vi "simple_strain_test.vi"() -> ()   [LabVIEW 2013]
uses:
  ctl/force_sensor_data.ctl
  ctl/strain_ctl.ctl
  <vilib>/Analysis/baseanly.llb/Mean (DBL).vi
  Global.vi
  <vilib>/Waveform/WDTFileIO.llb/ Write Waveform to File.vi
  <vilib>/Analysis/NI_AALBase.lvlib
panel:
  in  "정지":bool
  in  "탭 컨트롤 2":enum32{"페이지 1", "페이지 2"}(tab)
  out "ratio chart":T1(graph)
  out "balance ok":bool
  out "balance graph":T2(graph)
  out "Force Graph":waveform(dbl)[](graph)
  out "p 4":dbl format="%.2f"
  out "p 3":dbl format="%.2f"
  out "p 2":dbl format="%.2f"
  out "p 1":dbl format="%.2f"
  out "chart":dbl(graph)
  out "출력 클러스터":T3 {"mean" format="%.6f"; "mean" format="%.6f"; "mean" format="%.6f"; "mean" format="%.6f"}
  in  "cal":bool
  out "strain sum 2":dbl format="%.6f"
  out "strain sum1":dbl format="%.6f"
  out "g weight":dbl format="%0.2f"
  out "portion ok":bool
  in  "balance update":bool
  out "웨이브폼 그래프":dbl[][](graph)
  out "error out 2":errorcluster caption="error out"
  in  "Force Sensor data":T4 {"strain map"."x" format="%#.7f"}
  in  "write\nforce data":bool
  in  "탭 컨트롤":enum32{"페이지 1", "페이지 2"}(tab)
  in  "file path (dialog if empty)":path caption="파일 경로(비었을 경우 대화 상자 창)"
  out "숫자형":i32
  in  "save?":bool
  in  "filter":bool
  in  "Lower Cut-Off":dbl=100.0 caption="하위 컷오프"
  out "Strain_offset_data":waveform(dbl)[](array[waveform])
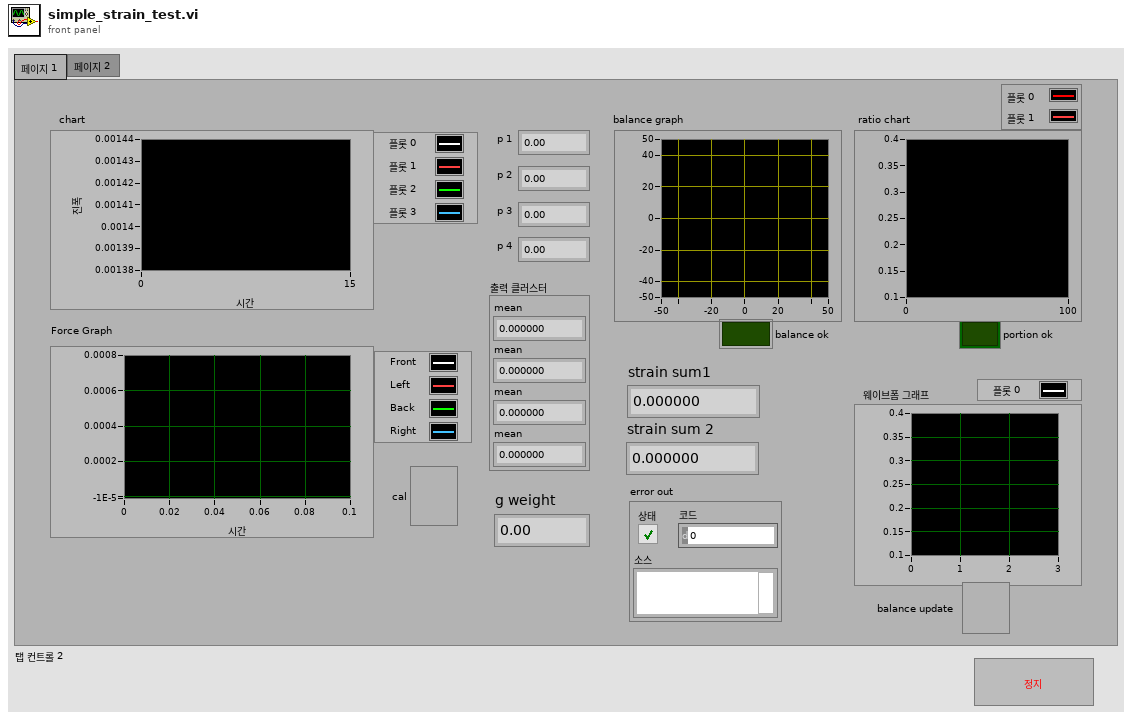
[diagram p1: front panel]
types:
  T1 = cluster{"[0]":dbl, "[1]":dbl, "[2]":dbl, "[3]":dbl, "[4]":dbl, "[5]":dbl, "[6]":dbl, "[7]":dbl, "[8]":dbl}
  T2 = cluster{"Balance xy wfs":cluster{"X":dbl, "Y":dbl}[]}[]
  T3 = cluster{"mean":dbl, "mean":dbl, "mean":dbl, "mean":dbl}
  T4 = typedef "force_sensor_data.ctl" = cluster{"weight":cluster{"front":dbl, "left":dbl, "back":dbl, "right":dbl}, "strain map":cluster{"x":dbl, "y":dbl}[]}
  T5 = typedef "strain_ctl.ctl" = enum16{"config", "start", "read", "close"}
  T6 = cluster{"Balance xy wfs":cluster{"X":dbl, "Y":dbl}[]}
  T7 = cluster{"[0]":dbl, "[1]":dbl, "[2]":dbl, "[3]":dbl}
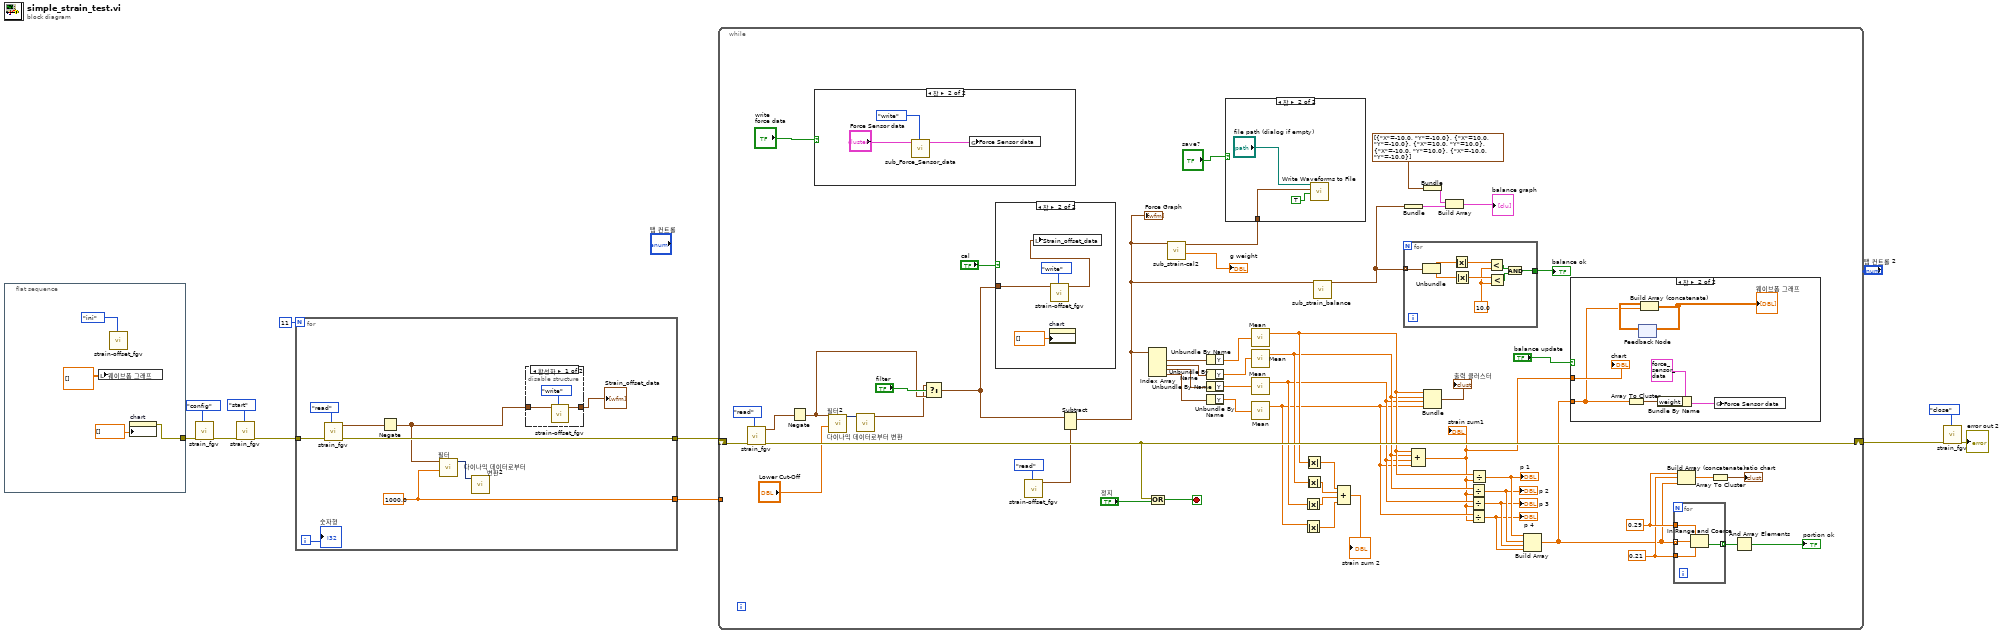
[diagram p0: block diagram]
diagram:
  n1 = flat-sequence {
    tunnel: [w15] -> w3
    frame #0 {
      n2 = local write "웨이브폼 그래프"(dbl[][] [] ("웨이브폼 그래프")) -> ()
      n3 = call "strain-offset_fgv.vi"("cmd"=enum16{"ini", "write", "read"}."ini") -> ()  [unwired: 9 in, 2 out]
      n4 = property on="chart" class="WFChart (엄격한)"("History Data"=dbl[] [] ("히스토리 데이터")) -> (error out=w15:errorcluster)  [unwired: 2 in, 1 out]
    }
  }
  n5 = call "strain_fgv.vi"("cmd"=strain_ctl."config", "error in"=w3) -> ("error out"=w7:errorcluster)  [unwired: 8 in, 1 out]
  n6 = call "strain_fgv.vi"("cmd"=strain_ctl."start", "error in"=w7) -> ("error out"=w6:errorcluster)  [unwired: 8 in, 1 out]
  n7 = for {
    N: 11 -> [_]
    tunnel: w6 -> [w24]
    tunnel: [w23] -> w5
    tunnel: [w20] -> w4
    i -> [w17]
    w20 = 1000.0 ("Lower Cut-Off")
    n8 = call "strain_fgv.vi"("cmd"=strain_ctl."read", "error in"=w24) -> ("error out"=w23:errorcluster, "data"=w21:waveform(dbl)[])  [unwired: 8 in]
    n9 = Negate(x=w21) -> (-x=w16:waveform(dbl)[])
    n10 = call "필터"("Lower Cut-Off"=w20, "Signal"=w16) -> ("Filtered Signal"=w22:dynamicdata)  [unwired: 8 in, 1 out]
    n11 = call "다이나믹 데이터로부터 변환2"("Dynamic Data Type"=w22) -> ()  [unwired: 3 in, 1 out]
    n12 = disable-structure shown="활성화" {
      disable-tunnel: w16 -> [w27 w28]
      disable-tunnel: [w26 w28] -> w19
      frame Enabled {
        n13 = call "strain-offset_fgv.vi"("cmd"=enum16{"ini", "write", "read"}."write", "data"=w27) -> ("Strain_offset_data"=w26:waveform(dbl)[])  [unwired: 8 in, 1 out]
      }
      frame Disabled {
      }
    }
    "Strain_offset_data" <- w19
    "숫자형" <- w17
  }
  n14 = while {
    shift-right: [w82] -> w11
    shift-left: w5 -> [w84]
    tunnel: w4 -> [_]
    stop <- w83 stop-if-true
    w37 = 0.21 ("하위 리미트")
    w38 = 0.29 ("하위 리미트")
    n15 = call "strain_fgv.vi"("cmd"=strain_ctl."read", "error in"=w84) -> ("error out"=w82:errorcluster, "data"=w69:waveform(dbl)[])  [unwired: 8 in]
    n16 = Negate(x=w69) -> (-x=w60:waveform(dbl)[])
    n17 = case shown="참" "write\nforce data" {
      frame False {
      }
      frame True {
        n18 = call "sub_Force_Sensor_data.vi"("cmd"=enum16{"write", "read"}."write", "Force Sensor data"="Force Sensor data") -> ("Force Sensor data out"=w107:T4)  [unwired: 9 in]
        n19 = global write "Global.vi" "Force Sensor data"(w107) -> ()
      }
    }
    n20 = call "필터2"("Lower Cut-Off"="Lower Cut-Off", "Signal"=w60) -> ("Filtered Signal"=w72:dynamicdata)  [unwired: 8 in, 1 out]
    n21 = call "다이나믹 데이터로부터 변환"("Dynamic Data Type"=w72) -> ("Array of Waveform"=w59:waveform(dbl)[])  [unwired: 3 in]
    n22 = Select(t=w59, s="filter", f=w60) -> (s? t:f=w63:waveform(dbl)[])
    n23 = case shown="참" "cal" {
      tunnel: w63 -> [_ w115]
      frame False {
      }
      frame True {
        n24 = property on="chart" class="WFChart (엄격한)"("History Data"=dbl[] [] ("히스토리 데이터")) -> ()  [unwired: 2 in, 2 out]
        n25 = call "strain-offset_fgv.vi"("cmd"=enum16{"ini", "write", "read"}."write", "data"=w115) -> ("Strain_offset_data"=w114:waveform(dbl)[])  [unwired: 8 in, 1 out]
        n26 = local write "Strain_offset_data"(w114) -> ()
      }
    }
    n27 = call "strain-offset_fgv.vi"("cmd"=enum16{"ini", "write", "read"}."read") -> ("Strain_offset_data"=w70:waveform(dbl)[])  [unwired: 9 in, 1 out]
    n28 = Subtract(1:w70, 2:w63) -> (0:w49:waveform(dbl)[])  [unwired: 1 in, 1 out]
    "Force Graph" <- w49
    n29 = Index Array(array=w49) -> (element #1=w80:waveform(dbl), element #2=w79:waveform(dbl), element #3=w78:waveform(dbl), element #4=w77:waveform(dbl))  [unwired: 4 in]
    n30 = Compound Arithmetic op=OR(w82, "정지") -> (w83:bool)
    n31 = call "sub_strain-cal2.vi"("strain wfs"=w49) -> ("force"=→"g weight":dbl, "force wf"=w65:waveform(dbl))  [unwired: 9 in]
    n32 = Unbundle By Name(w80) -> ("Y"=w76:dbl[])
    n33 = Unbundle By Name(w79) -> ("Y"=w73:dbl[])
    n34 = Unbundle By Name(w78) -> ("Y"=w74:dbl[])
    n35 = Unbundle By Name(w77) -> ("Y"=w75:dbl[])
    n36 = case shown="참" "save?" {
      tunnel: w65 -> [_ w111]
      frame False {
      }
      frame True {
        n37 = call-poly <vilib>:"Write Waveforms to File.vi"("append to file? (new file:F)"=TRUE, "waveform"=w111, "file path (dialog if empty)"="file path (dialog if empty)") -> ()  [unwired: 7 in, 2 out]
      }
    }
    n38 = call-poly <vilib>:"Mean.vi"("X"=w76) -> ("mean"=w57:dbl)  [unwired: 1 out]
    n39 = call-poly <vilib>:"Mean.vi"("X"=w73) -> ("mean"=w56:dbl)  [unwired: 1 out]
    n40 = call-poly <vilib>:"Mean.vi"("X"=w74) -> ("mean"=w55:dbl)  [unwired: 1 out]
    n41 = call-poly <vilib>:"Mean.vi"("X"=w75) -> ("mean"=w54:dbl)  [unwired: 1 out]
    n42 = Absolute Value(x=w55) -> (abs(x)=w50:dbl)
    n43 = Absolute Value(x=w54) -> (abs(x)=w53:dbl)
    n44 = Absolute Value(x=w57) -> (abs(x)=w52:dbl)
    n45 = Absolute Value(x=w56) -> (abs(x)=w51:dbl)
    n46 = call "sub_strain_balance.vi"("strain_offset_wf"=w49) -> ("Balance xy wfs"=w32:cluster{"X":dbl, "Y":dbl}[])  [unwired: 9 in, 1 out]
    n47 = Compound Arithmetic op=ADD(w52, w51, w50, w53) -> (→"strain sum 2":dbl)
    n48 = for {
      tunnel: w32 -> [w105] mode=indexing
      tunnel: [w97] -> w45
      w100 = 10.0 ("Y")
      n49 = Unbundle(w105) -> ("X"=w103:dbl, "Y"=w104:dbl)
      n50 = Absolute Value(x=w103) -> (abs(x)=w102:dbl)
      n51 = Absolute Value(x=w104) -> (abs(x)=w101:dbl)
      n52 = Less?(x=w102, y=w100) -> (x < y?=w98:bool)
      n53 = Less?(x=w101, y=w100) -> (x < y?=w99:bool)
      n54 = And(x=w98, y=w99) -> (x .and. y?=w97:bool)
    }
    "balance ok" <- w45
    n55 = Bundle("Balance xy wfs"=w32) -> (w31:T6)  [unwired: 1 in]
    n56 = Compound Arithmetic op=ADD(w57, w56, w55, w54) -> (w30:dbl)
    "strain sum1" <- w30
    n57 = Bundle("Balance xy wfs"=cluster{"X":dbl, "Y":dbl}[] [{"X"=-10.0, "Y"=-10.0}, {"X"=10.0, "Y"=-10.0}, {"X"=10.0, "Y"=10.0}, {"X"=-10.0, "Y"=10.0}, {"X"=-10.0, "Y"=-10.0}]) -> (w46:T6)  [unwired: 1 in]
    n58 = Bundle("mean"=w57, "mean"=w56, "mean"=w55, "mean"=w54) -> (→"출력 클러스터":T3)  [unwired: 1 in]
    n59 = Build Array(w46, w31) -> (→"balance graph":T2)
    n60 = Divide(x=w56, y=w30) -> (x/y=w43:dbl)
    "p 2" <- w43
    n61 = Divide(x=w55, y=w30) -> (x/y=w42:dbl)
    "p 3" <- w42
    n62 = Divide(x=w54, y=w30) -> (x/y=w41:dbl)
    "p 4" <- w41
    n63 = Divide(x=w57, y=w30) -> (x/y=w44:dbl)
    "p 1" <- w44
    n64 = Build Array(w44, w43, w42, w41) -> (w33:dbl[])
    n65 = case shown="참" "balance update" {
      tunnel: w33 -> [_ w86]
      tunnel: w30 -> [_ w88]
      frame False {
      }
      frame True {
        n66 = Array To Cluster(array=w86) -> (cluster=w92:T7)
        n67 = feedback #1() -> (w87:dbl[][])  [unwired: 1 in]
        n68 = Build Array (concatenate)(w87, w86) -> (w89:dbl[][])
        "웨이브폼 그래프" <- w89
        n69 = feedback-in #1(w89) -> ()
        n70 = Bundle By Name(cluster=T4 {"weight"={"front"=0.26, "left"=0.18, "back"=0.3, "right"=0.26}, "strain map"=[{"x"=-7.5e-05, "y"=-80.0}, {"x"=-5.7e-05, "y"=-60.61}, {"x"=-4.5e-05, "y"=-50.0}, {"x"=0.0, "y"=0.0}, {"x"=4.5e-05, "y"=50.0}, {"x"=5.7e-05, "y"=60.61}, {"x"=7.5e-05, "y"=80.0}, {"x"=0.000106, "y"=110.0}, {"x"=0.000243, "y"=260.0}, {"x"=0.00047, "y"=512.0}, {"x"=0.000718, "y"=878.0}, {"x"=0.00088, "y"=1042.0}, {"x"=0.00116, "y"=1395.0}, {"x"=0.00156, "y"=2090.0}]} ("Force Sensor data"), "weight"=w92) -> (w90:T4)
        n71 = global write "Global.vi" "Force Sensor data"(w90) -> ()
        "chart" <- w88
      }
    }
    n72 = for {
      tunnel: w33 -> [w96] mode=indexing
      tunnel: [w95] -> w40 mode=indexing
      tunnel: w37 -> [w94]
      tunnel: w38 -> [w93]
      n73 = In Range and Coerce(upper limit=w93, x=w96, lower limit=w94) -> (In Range?=w95:bool)  [unwired: 1 out]
    }
    n74 = Build Array (concatenate)(w38, w37, w33) -> (w36:dbl[])
    n75 = Array To Cluster(array=w36) -> (cluster=→"ratio chart":T1)
    n76 = And Array Elements(Boolean array=w40) -> (logical AND=→"portion ok":bool)
  }
  n77 = call "strain_fgv.vi"("cmd"=strain_ctl."close", "error in"=w11) -> ("error out"=→"error out 2":errorcluster)  [unwired: 8 in, 1 out]
